vi "InitializeDetectionAgent.vi"() -> (0 "error out":errorcluster, 1 "Object Tracking Session Out":T3, 2 "Session Out":T2, 3 "connection ID":refnum<k5>, 4 "Aquisition Image":T1)   [LabVIEW 2019]
uses:
  <vilib>/vision/Tracking.llb/IMAQ Object Tracking Session.ctl
  <vilib>/userdefined/High Color/IMAQdx.ctl
  <vilib>/vision/Image Controls.llb/IMAQ Image.ctl
  <vilib>/Utility/config.llb/Read Key (String).vi
  <vilib>/Utility/config.llb/Read Key (U32).vi
  <vilib>/vision/driver/NI_Vision_Acquisition_Software.lvlib
  <resource>/objmgr/imaqdx.rc
  <vilib>/Utility/config.llb/NI_LVConfig.lvlib
panel:
  in  "Percent of Images Reserved by Driver":dbl=50.0
  in  "Overwrite Mode":u16(ring) items=["Get Oldest"=0, "Fail"=2, "Get Newest"=3]
  in  "Number of Images":u32=10
  in  "Camera Name":refnum<k21>="cam0" caption="IMAQdx Session"
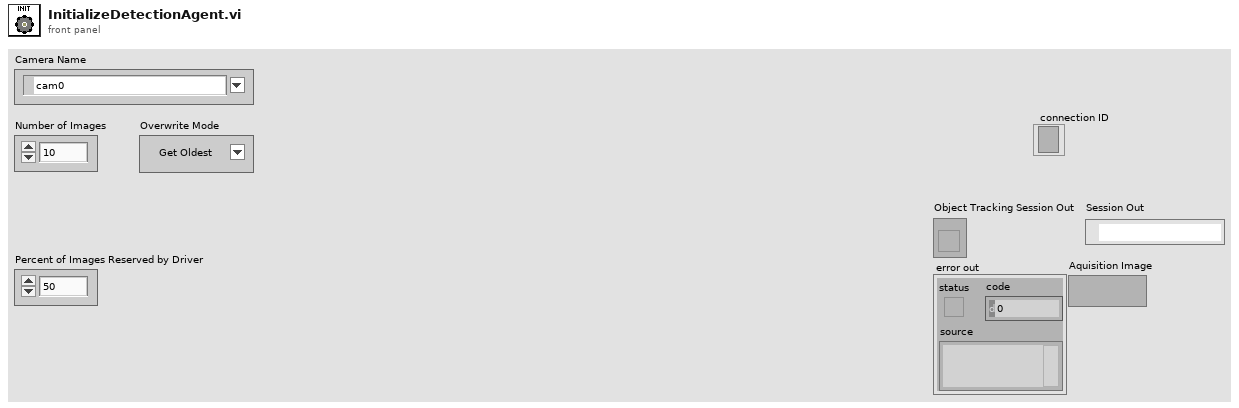
[diagram p1: front panel]
types:
  T1 = typedef "IMAQ Image.ctl" = refnum<image>
  T2 = typedef "IMAQdx.ctl" = refnum<k21>
  T3 = typedef "IMAQ Object Tracking Session.ctl" = refnum<k20>
  T4 = cluster{"Number of Histogram Bins":i32, "Blending Parameter (%)":dbl, "Maximum Iterations":i32}
  T5 = typedef "Image Type" = u32
  T6 = typedef "NI_LVConfig.lvlib/Config Data RefNum.ctl" = refnum<k1>
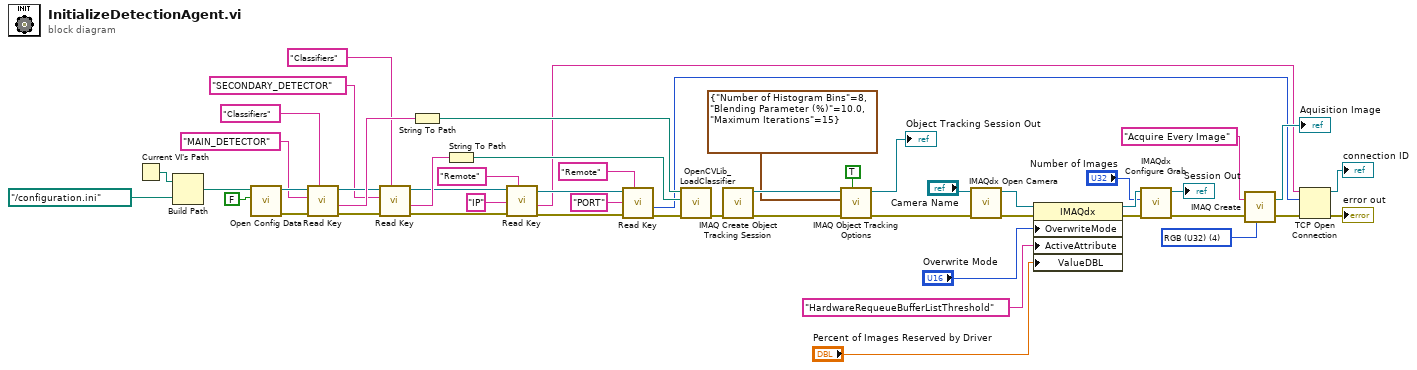
[diagram p0: block diagram]
diagram:
  w40 = T5 4 items=["Grayscale (U8)", "Grayscale (I16)", "Grayscale (SGL)", "Complex (CSG)", "RGB (U32)", "HSL (U32)", "RGB (U64)", "Grayscale (U16)"] ("Image Type")
  n1 = Current VI's Path() -> (path=w23:path)
  n2 = Build Path(base path=w23, name or relative path=path "../configuration.ini" ("Face Cascade Path")) -> (appended path=w21:path)
  n3 = call <vilib>:"Open Config Data.vi"("create file if necessary (T)"=FALSE, "configuration file path"=w21) -> ("error out"=w26:errorcluster, "refnum"=w27:T6)  [unwired: 7 in, 1 out]
  n4 = call-poly <vilib>:"Read Key.vi"("section"="Classifiers", "error in (no error)"=w26, "key"="MAIN_DETECTOR", "refnum"=w27) -> ("error out"=w12:errorcluster, "value"=w19:string, "refnum out"=w17:T6)  [unwired: 4 in, 1 out]
  n5 = call-poly <vilib>:"Read Key.vi"("section"="Classifiers", "error in (no error)"=w12, "key"="SECONDARY_DETECTOR", "refnum"=w17) -> ("error out"=w10:errorcluster, "value"=w14:string, "refnum out"=w11:T6)  [unwired: 4 in, 1 out]
  n6 = String To Path(string=w19) -> (path=w18:path)
  n7 = String To Path(string=w14) -> (path=w13:path)
  n8 = call-poly <vilib>:"Read Key.vi"("section"="Remote", "error in (no error)"=w10, "key"="IP", "refnum"=w11) -> ("error out"=w8:errorcluster, "value"=w7:string, "refnum out"=w9:T6)  [unwired: 4 in, 1 out]
  n9 = call-poly <vilib>:"Read Key.vi"("section"="Remote", "error in (no error)"=w8, "key"="PORT", "refnum"=w9) -> ("error out"=w5:errorcluster, "value"=w6:u32)  [unwired: 4 in, 2 out]
  n10 = call "OpenCVLib_LoadClassifier.vi"("error in (no error)"=w5, "faceCheckerCascadePath"=w13, "faceCascadePath"=w18) -> ("error out"=w33:errorcluster)  [unwired: 8 in]
  n11 = call "IMAQ Create Object Tracking Session"("error in (no error)"=w33) -> ("error out"=w37:errorcluster, "Object Tracking Session"=w39:T3)  [unwired: 9 out]
  n12 = call-poly "IMAQ Object Tracking Options"("Get/Set (Get)"=TRUE, "error in (no error)"=w37, "Mean Shift Options in"=T4 {"Number of Histogram Bins"=8, "Blending Parameter (%)"=10.0, "Maximum Iterations"=15}, "Object Tracking Session In"=w39) -> ("error out"=w35:errorcluster, "Object Tracking Session Out"=→"Object Tracking Session Out":T3)  [unwired: 5 in, 1 out]
  n13 = call <vilib>:"IMAQdx Open Camera.vi"("error in"=w35, "Session In"="Camera Name") -> ("error out"=w49:errorcluster, "Session Out"=w50:T2)  [unwired: 1 in, 7 out]
  n14 = property class="IMAQdx"(reference=w50, error in=w49, "OverwriteMode"="Overwrite Mode", "ActiveAttribute"="HardwareRequeueBufferListThreshold", "ValueDBL"="Percent of Images Reserved by Driver") -> (reference out=w43:T2, error out=w42:errorcluster)
  n15 = call <vilib>:"IMAQdx Configure Grab.vi"("error in"=w42, "Number of Buffers"="Number of Images", "Session In"=w43) -> ("error out"=w30:errorcluster, "Session Out"=→"Session Out":T2)  [unwired: 7 in]
  n16 = call "IMAQ Create"("Image Name"="Acquire Every Image", "Image Type"=w40, "error in (no error)"=w30) -> ("New Image"=→"Aquisition Image":T1, "error out"=w29:errorcluster)  [unwired: 1 in, 1 out]
  n17 = TCP Open Connection(address=w7, remote port or service name=w6, error in (no error)=w29) -> (connection ID=→"connection ID":refnum<k5>, error out=→"error out":errorcluster)  [unwired: 2 in]
